vi "Adquisicio_projecte_InsEl (2).vi"() -> ()   [LabVIEW 2014]
uses:
  <vilib>/DAQmx/read.llb/DAQmx Read (Analog 1D Wfm NChan NSamp).vi
  <vilib>/DAQmx/configure/timing.llb/DAQmx Timing (Sample Clock).vi
  <vilib>/DAQmx/miscellaneous.llb/DAQmx Fill In Error Info.vi
panel:
  in  "T alarm max CH 4":dbl
  in  "T alarm min CH 4":dbl
  in  "T alarm max CH 3":dbl
  in  "T alarm min CH 3":dbl
  in  "T alarm min CH 2":dbl
  in  "T alarm max CH 2":dbl
  in  "T alarm max CH 1":dbl
  in  "T alarm min CH 1":dbl
  out "IND CH 4":u32(colorbox)
  out "IND CH 3":u32(colorbox)
  out "IND CH 2":u32(colorbox)
  out "IND CH 1":u32(colorbox)
  in  "V2":dbl
  in  "V1":dbl
  in  "T2":dbl
  in  "T1":dbl
  in  "Numero de Media":dbl
  in  "Durada adquisició(s)":dbl
  in  "Temps entre adquisicions(s)":dbl
  out "?":bool
  out "?":bool
  out "?":bool
  out "?":bool
  in  "CH 4":bool
  in  "CH 3":bool
  in  "CH 2":bool
  in  "CH 1":bool
  in  "?":bool
  in  "?":bool
  out "Registro Temperatura CH 4":dbl(graph)
  out "Registro Temperatura CH 3":dbl(graph)
  out "Registro Temperatura CH 2":dbl(graph)
  out "Registro Temperatura CH 1":dbl(graph)
  in  "Tab Control":enum32{"CH 1", "CH 2", "CH 3", "CH 4"}(tab)
  out "T min CH 1":dbl
  out "T max CH 1":dbl
  out "Desviació 1":dbl
  out "H CH 1":dbl[](array[numeric])
  out "MEDIA CH 1":dbl
  out "Tiempo T max CH1":string
  out "Tiempo T min CH1":string
  out "H CH 2":dbl[](array[numeric])
  out "T max CH 2":dbl
  out "T min CH 2":dbl
  out "Desviació 2":dbl
  out "MEDIA CH 2":dbl
  out "Tiempo T max CH2":string
  out "Tiempo T min CH2":string
  out "H CH 3":dbl[](array[numeric])
  out "T max CH 3":dbl
  out "T min CH 3":dbl
  out "Desviació 3":dbl
  out "MEDIA CH 3":dbl
  out "Tiempo T max CH3":string
  out "Tiempo T min CH3":string
  out "H CH 4":dbl[](array[numeric])
  out "T max CH 4":dbl
  out "T min CH 4":dbl
  out "Desviació 4":dbl
  out "Tiempo T max CH4":string
  out "Tiempo T min CH4":string
  out "MEDIA CH 4":dbl
  # "SISTEMA D'ALARMES"
  # "ACTIVACIÓ CANALS"
  # "CONFIGURACIÓ"
  # "CALIBRATGE"
  # "Temperatura per sobre del màxim"
  # "Temperatura corecta"
  # "Temperatura per sota del mínim"
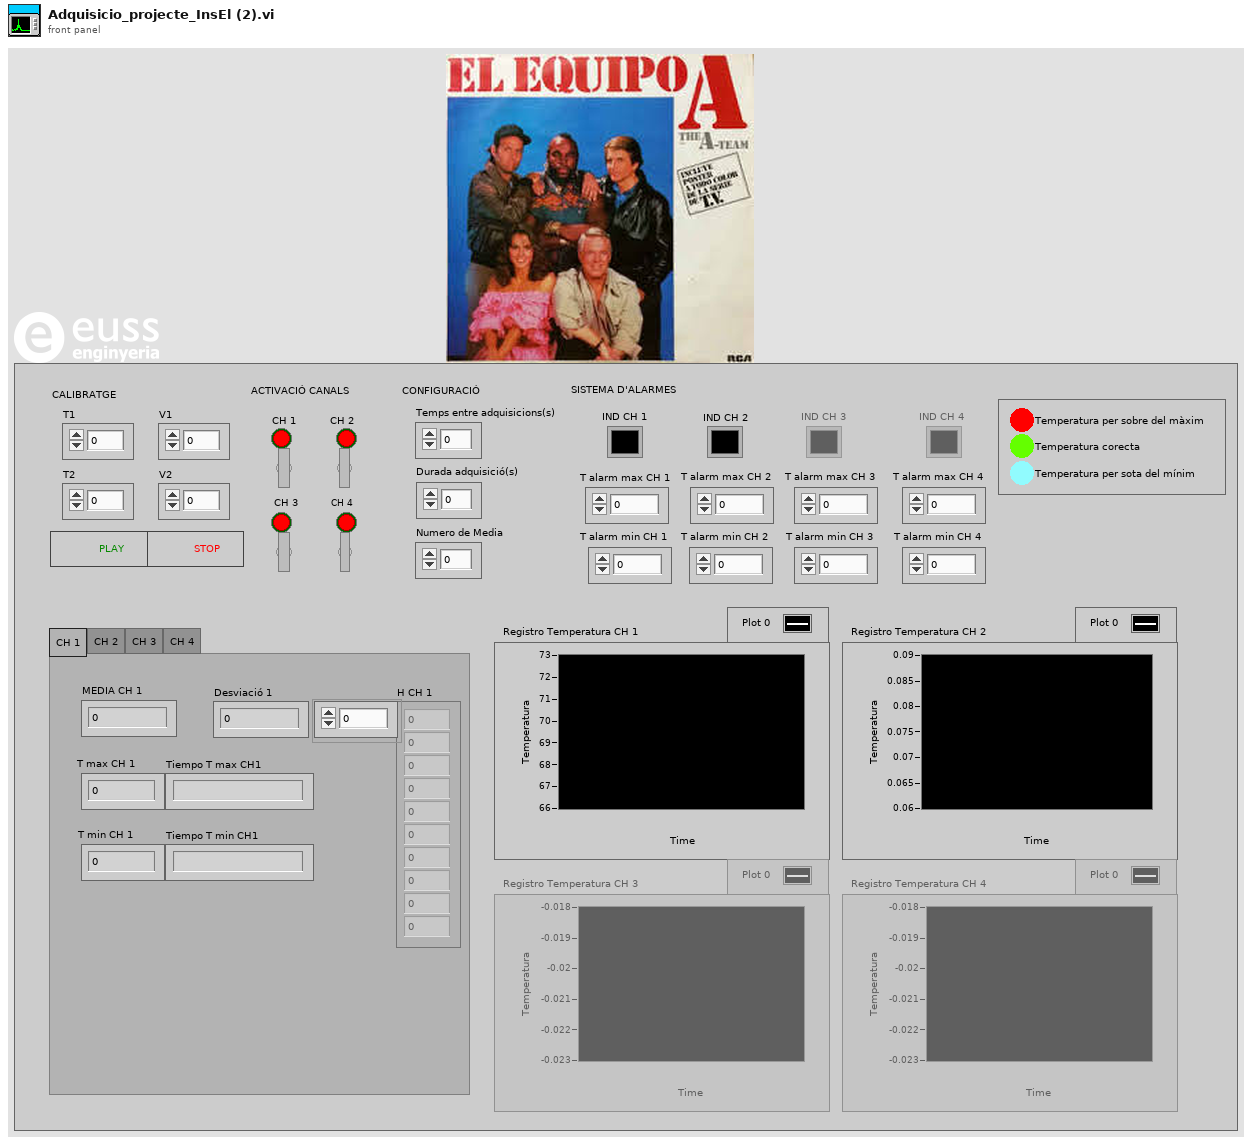
[diagram p1: front panel]
types:
  T1 = enum16{"open", "replace", "create", "open or create", "replace or create", "replace or create with confirmation"}
  T2 = enum8{"Enabled", "Disabled", "Disabled and Grayed Out"}
  T3 = cluster{"CH 1":bool, "CH 2":bool, "CH 3":bool, "CH 4":bool}
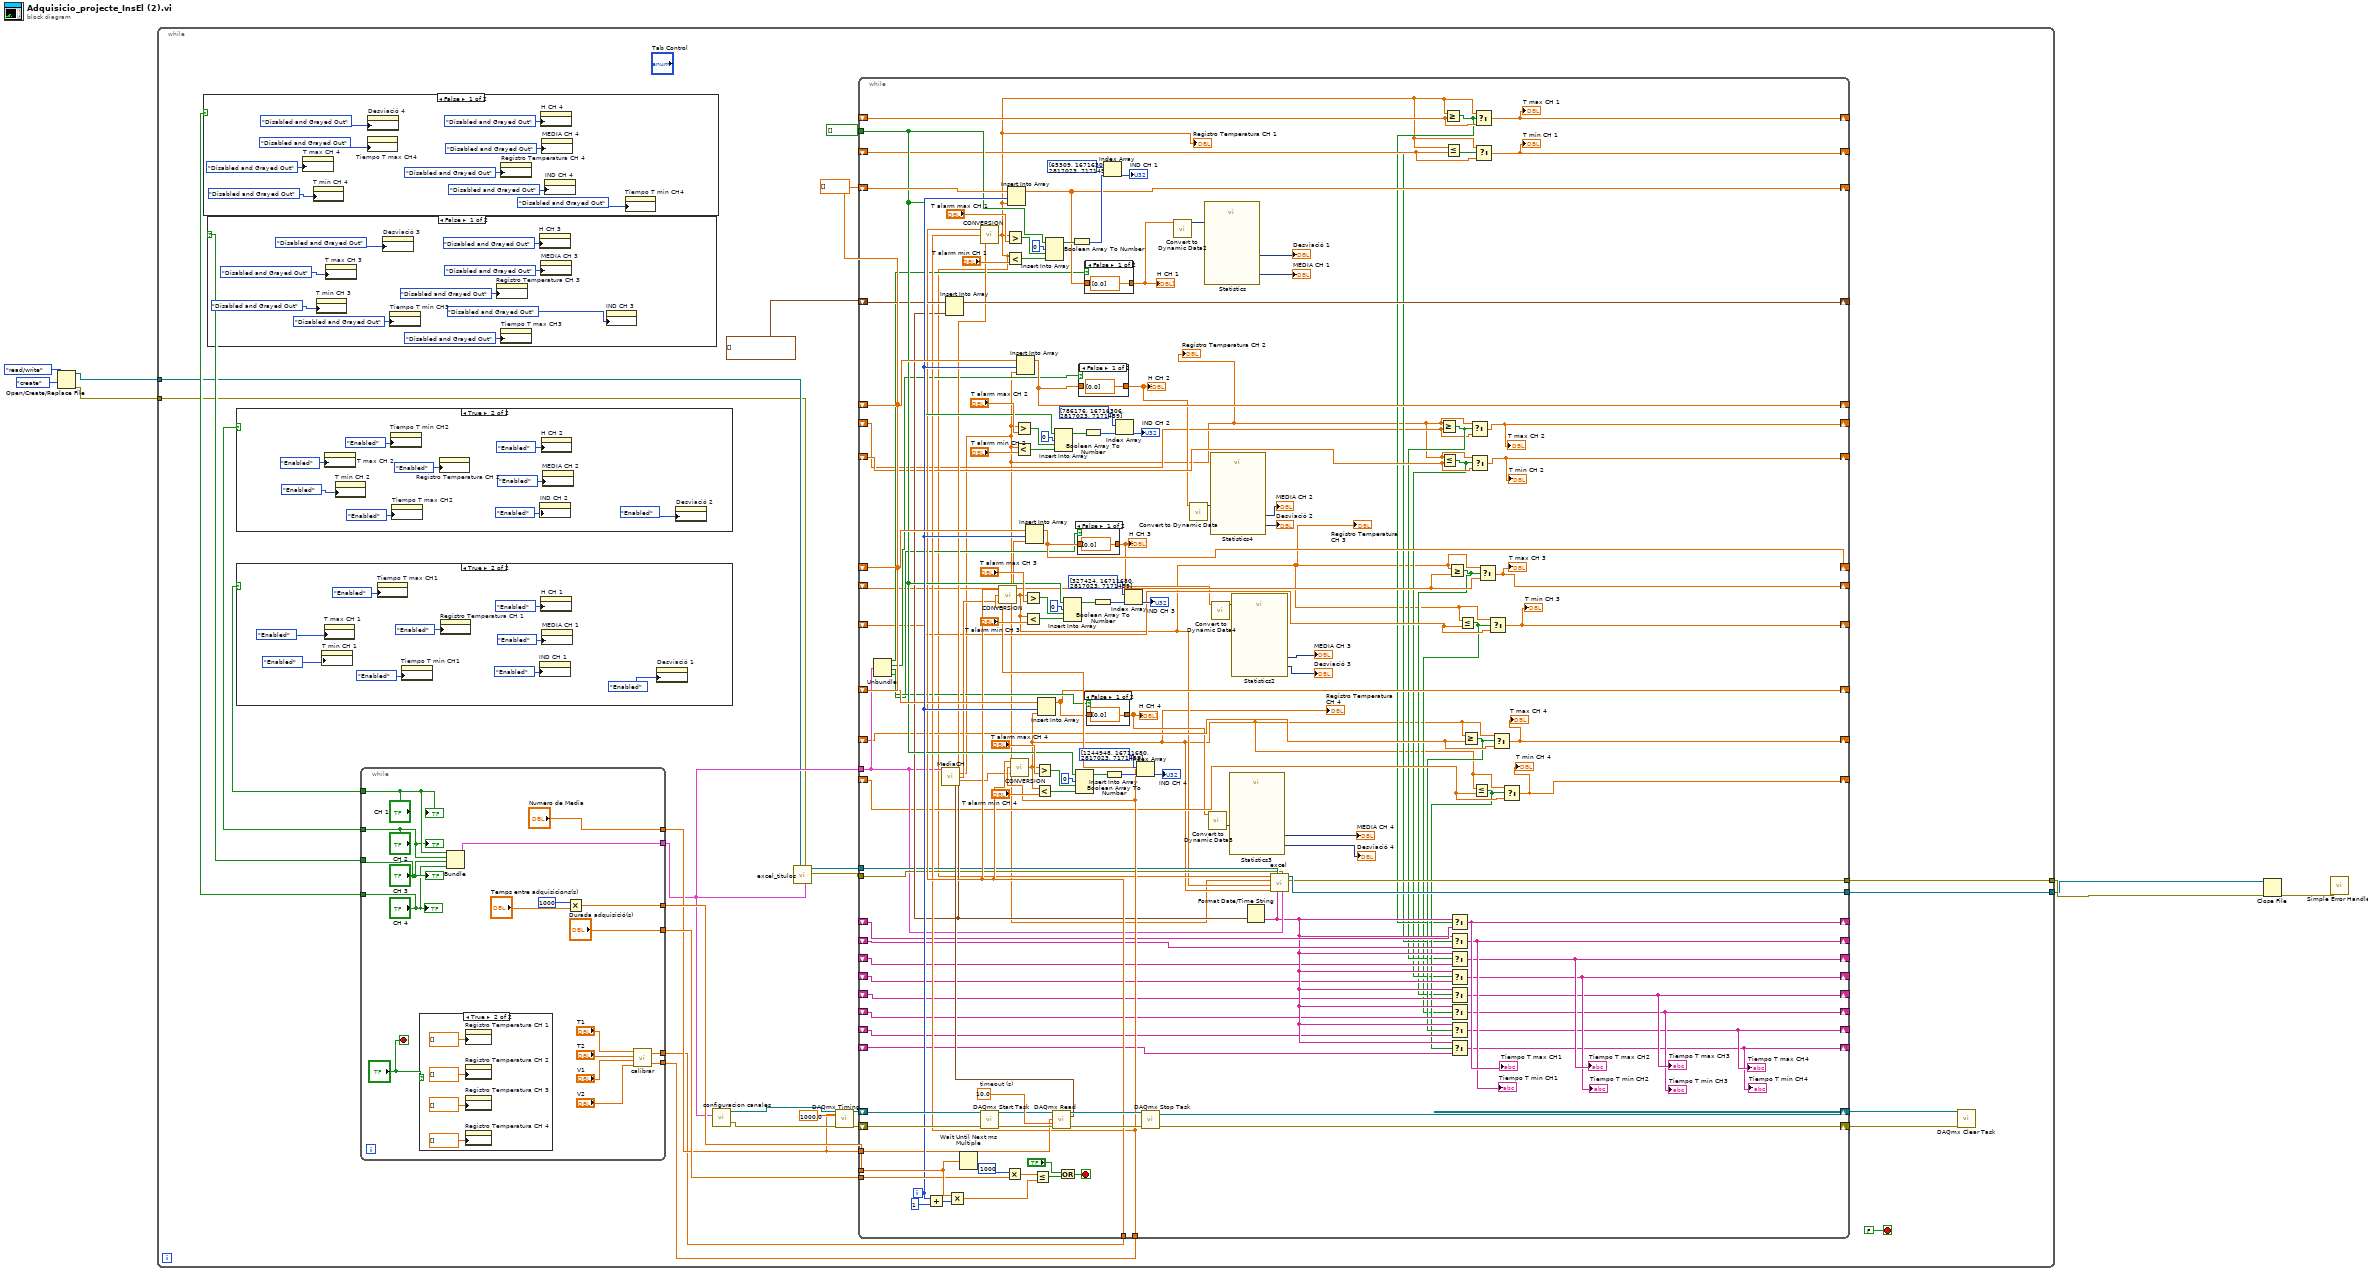
[diagram p0: block diagram]
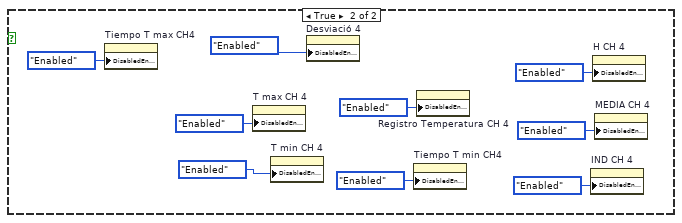
[diagram p2: hidden frame]
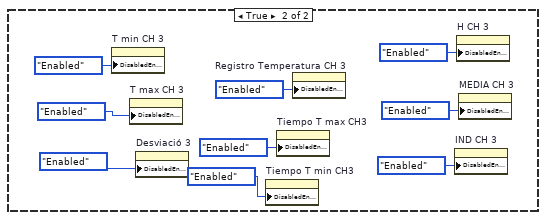
[diagram p3: hidden frame]
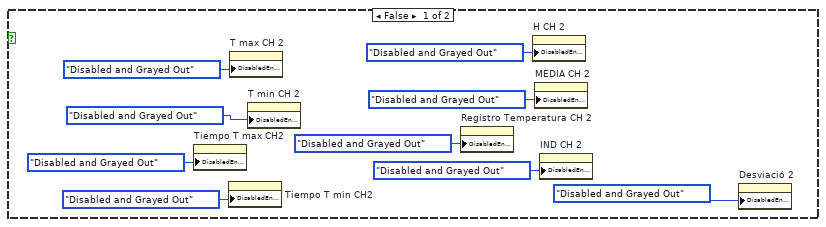
[diagram p4: hidden frame]
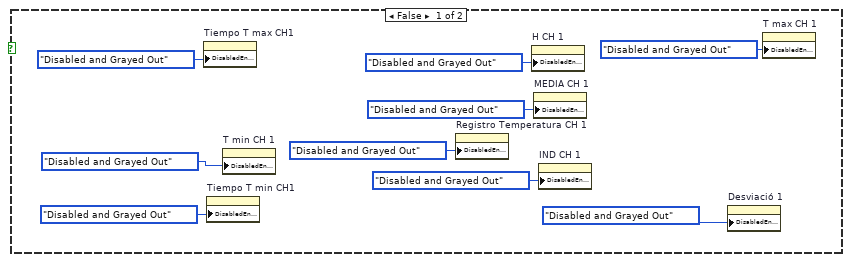
[diagram p5: hidden frame]
diagram:
  n1 = Open/Create/Replace File(operation (0:open)=T1."create", access (0:read/write)=enum16{"read/write", "read-only", "write-only"}."read/write") -> (refnum out=w5:refnum<file>, error out=w4:errorcluster)  [unwired: 4 in, 1 out]
  n2 = while {
    tunnel: w5 -> [w13]
    tunnel: w4 -> [w12]
    tunnel: [w10] -> w2
    tunnel: [w9] -> w1
    stop <- FALSE stop-if-true
    w28 = dbl[] [] ("array")
    n3 = while {
      tunnel: [w123] -> w14
      tunnel: ["CH 1"] -> w26
      tunnel: ["CH 2"] -> w23
      tunnel: ["CH 3"] -> w24
      tunnel: ["CH 4"] -> w25
      tunnel: ["Numero de Media"] -> w19
      tunnel: [w114] -> w21
      tunnel: ["Durada adquisició(s)"] -> w20
      tunnel: [w108] -> w18
      tunnel: [w107] -> w17
      stop <- "?" stop-if-true
      n4 = case shown="True" "?" {
        frame False {
        }
        frame True {
          n5 = property on="Registro Temperatura CH 1" class="WFChart (strict)"("History Data"=dbl[] []) -> ()  [unwired: 2 in, 2 out]
          n6 = property on="Registro Temperatura CH 2" class="WFChart (strict)"("History Data"=dbl[] []) -> ()  [unwired: 2 in, 2 out]
          n7 = property on="Registro Temperatura CH 3" class="WFChart (strict)"("History Data"=dbl[] []) -> ()  [unwired: 2 in, 2 out]
          n8 = property on="Registro Temperatura CH 4" class="WFChart (strict)"("History Data"=dbl[] []) -> ()  [unwired: 2 in, 2 out]
        }
      }
      n9 = Bundle("CH 1"="CH 1", "CH 2"="CH 2", "CH 3"="CH 3", "CH 4"="CH 4") -> (w123:T3)  [unwired: 1 in]
      n10 = Multiply(x=1000, y="Temps entre adquisicions(s)") -> (x*y=w114:dbl)
      n11 = call "calibrar.vi"("V 2"="V2", "V1"="V1", "Temp2"="T2", "Temp"="T1") -> ("B"=w107:dbl, "A"=w108:dbl)
      "?" <- "CH 1"
      "?" <- "CH 2"
      "?" <- "CH 3"
      "?" <- "CH 4"
    }
    n12 = case shown="False" w25 {
      frame False {
        n13 = property on="T max CH 4" class="DigNum (strict)"("DisabledEnum"=T2."Disabled and Grayed Out" ("Disabled")) -> ()  [unwired: 2 in, 2 out]
        n14 = property on="T min CH 4" class="DigNum (strict)"("DisabledEnum"=T2."Disabled and Grayed Out" ("Disabled")) -> ()  [unwired: 2 in, 2 out]
        n15 = property on="Tiempo T max CH4" class="Str"("DisabledEnum"=T2."Disabled and Grayed Out" ("Disabled")) -> ()  [unwired: 2 in, 2 out]
        n16 = property on="Desviació 4" class="DigNum (strict)"("DisabledEnum"=T2."Disabled and Grayed Out" ("Disabled")) -> ()  [unwired: 2 in, 2 out]
        n17 = property on="Registro Temperatura CH 4" class="WFChart (strict)"("DisabledEnum"=T2."Disabled and Grayed Out" ("Disabled")) -> ()  [unwired: 2 in, 2 out]
        n18 = property on="H CH 4" class="Arr (strict)"("DisabledEnum"=T2."Disabled and Grayed Out" ("Disabled")) -> ()  [unwired: 2 in, 2 out]
        n19 = property on="MEDIA CH 4" class="DigNum (strict)"("DisabledEnum"=T2."Disabled and Grayed Out" ("Disabled")) -> ()  [unwired: 2 in, 2 out]
        n20 = property on="IND CH 4" class="ColBox"("DisabledEnum"=T2."Disabled and Grayed Out" ("Disabled")) -> ()  [unwired: 2 in, 2 out]
        n21 = property on="Tiempo T min CH4" class="Str"("DisabledEnum"=T2."Disabled and Grayed Out" ("Disabled")) -> ()  [unwired: 2 in, 2 out]
      }
      frame True {
        n22 = property on="Tiempo T max CH4" class="Str"("DisabledEnum"=T2."Enabled" ("Disabled")) -> ()  [unwired: 2 in, 2 out]
        n23 = property on="T max CH 4" class="DigNum (strict)"("DisabledEnum"=T2."Enabled" ("Disabled")) -> ()  [unwired: 2 in, 2 out]
        n24 = property on="T min CH 4" class="DigNum (strict)"("DisabledEnum"=T2."Enabled" ("Disabled")) -> ()  [unwired: 2 in, 2 out]
        n25 = property on="Desviació 4" class="DigNum (strict)"("DisabledEnum"=T2."Enabled" ("Disabled")) -> ()  [unwired: 2 in, 2 out]
        n26 = property on="Tiempo T min CH4" class="Str"("DisabledEnum"=T2."Enabled" ("Disabled")) -> ()  [unwired: 2 in, 2 out]
        n27 = property on="Registro Temperatura CH 4" class="WFChart (strict)"("DisabledEnum"=T2."Enabled" ("Disabled")) -> ()  [unwired: 2 in, 2 out]
        n28 = property on="IND CH 4" class="ColBox"("DisabledEnum"=T2."Enabled" ("Disabled")) -> ()  [unwired: 2 in, 2 out]
        n29 = property on="H CH 4" class="Arr (strict)"("DisabledEnum"=T2."Enabled" ("Disabled")) -> ()  [unwired: 2 in, 2 out]
        n30 = property on="MEDIA CH 4" class="DigNum (strict)"("DisabledEnum"=T2."Enabled" ("Disabled")) -> ()  [unwired: 2 in, 2 out]
      }
    }
    n31 = case shown="False" w24 {
      frame False {
        n32 = property on="T min CH 3" class="DigNum (strict)"("DisabledEnum"=T2."Disabled and Grayed Out" ("Disabled")) -> ()  [unwired: 2 in, 2 out]
        n33 = property on="T max CH 3" class="DigNum (strict)"("DisabledEnum"=T2."Disabled and Grayed Out" ("Disabled")) -> ()  [unwired: 2 in, 2 out]
        n34 = property on="Desviació 3" class="DigNum (strict)"("DisabledEnum"=T2."Disabled and Grayed Out" ("Disabled")) -> ()  [unwired: 2 in, 2 out]
        n35 = property on="Tiempo T min CH3" class="Str"("DisabledEnum"=T2."Disabled and Grayed Out" ("Disabled")) -> ()  [unwired: 2 in, 2 out]
        n36 = property on="Registro Temperatura CH 3" class="WFChart (strict)"("DisabledEnum"=T2."Disabled and Grayed Out" ("Disabled")) -> ()  [unwired: 2 in, 2 out]
        n37 = property on="Tiempo T max CH3" class="Str"("DisabledEnum"=T2."Disabled and Grayed Out" ("Disabled")) -> ()  [unwired: 2 in, 2 out]
        n38 = property on="H CH 3" class="Arr (strict)"("DisabledEnum"=T2."Disabled and Grayed Out" ("Disabled")) -> ()  [unwired: 2 in, 2 out]
        n39 = property on="MEDIA CH 3" class="DigNum (strict)"("DisabledEnum"=T2."Disabled and Grayed Out" ("Disabled")) -> ()  [unwired: 2 in, 2 out]
        n40 = property on="IND CH 3" class="ColBox"("DisabledEnum"=T2."Disabled and Grayed Out" ("Disabled")) -> ()  [unwired: 2 in, 2 out]
      }
      frame True {
        n41 = property on="T min CH 3" class="DigNum (strict)"("DisabledEnum"=T2."Enabled" ("Disabled")) -> ()  [unwired: 2 in, 2 out]
        n42 = property on="T max CH 3" class="DigNum (strict)"("DisabledEnum"=T2."Enabled" ("Disabled")) -> ()  [unwired: 2 in, 2 out]
        n43 = property on="Desviació 3" class="DigNum (strict)"("DisabledEnum"=T2."Enabled" ("Disabled")) -> ()  [unwired: 2 in, 2 out]
        n44 = property on="Tiempo T min CH3" class="Str"("DisabledEnum"=T2."Enabled" ("Disabled")) -> ()  [unwired: 2 in, 2 out]
        n45 = property on="Tiempo T max CH3" class="Str"("DisabledEnum"=T2."Enabled" ("Disabled")) -> ()  [unwired: 2 in, 2 out]
        n46 = property on="Registro Temperatura CH 3" class="WFChart (strict)"("DisabledEnum"=T2."Enabled" ("Disabled")) -> ()  [unwired: 2 in, 2 out]
        n47 = property on="IND CH 3" class="ColBox"("DisabledEnum"=T2."Enabled" ("Disabled")) -> ()  [unwired: 2 in, 2 out]
        n48 = property on="H CH 3" class="Arr (strict)"("DisabledEnum"=T2."Enabled" ("Disabled")) -> ()  [unwired: 2 in, 2 out]
        n49 = property on="MEDIA CH 3" class="DigNum (strict)"("DisabledEnum"=T2."Enabled" ("Disabled")) -> ()  [unwired: 2 in, 2 out]
      }
    }
    n50 = case shown="True" w23 {
      frame False {
        n51 = property on="Tiempo T max CH2" class="Str"("DisabledEnum"=T2."Disabled and Grayed Out" ("Disabled")) -> ()  [unwired: 2 in, 2 out]
        n52 = property on="Tiempo T min CH2" class="Str"("DisabledEnum"=T2."Disabled and Grayed Out" ("Disabled")) -> ()  [unwired: 2 in, 2 out]
        n53 = property on="T max CH 2" class="DigNum (strict)"("DisabledEnum"=T2."Disabled and Grayed Out" ("Disabled")) -> ()  [unwired: 2 in, 2 out]
        n54 = property on="T min CH 2" class="DigNum (strict)"("DisabledEnum"=T2."Disabled and Grayed Out" ("Disabled")) -> ()  [unwired: 2 in, 2 out]
        n55 = property on="Registro Temperatura CH 2" class="WFChart (strict)"("DisabledEnum"=T2."Disabled and Grayed Out" ("Disabled")) -> ()  [unwired: 2 in, 2 out]
        n56 = property on="H CH 2" class="Arr (strict)"("DisabledEnum"=T2."Disabled and Grayed Out" ("Disabled")) -> ()  [unwired: 2 in, 2 out]
        n57 = property on="MEDIA CH 2" class="DigNum (strict)"("DisabledEnum"=T2."Disabled and Grayed Out" ("Disabled")) -> ()  [unwired: 2 in, 2 out]
        n58 = property on="IND CH 2" class="ColBox"("DisabledEnum"=T2."Disabled and Grayed Out" ("Disabled")) -> ()  [unwired: 2 in, 2 out]
        n59 = property on="Desviació 2" class="DigNum (strict)"("DisabledEnum"=T2."Disabled and Grayed Out" ("Disabled")) -> ()  [unwired: 2 in, 2 out]
      }
      frame True {
        n60 = property on="T max CH 2" class="DigNum (strict)"("DisabledEnum"=T2."Enabled" ("Disabled")) -> ()  [unwired: 2 in, 2 out]
        n61 = property on="T min CH 2" class="DigNum (strict)"("DisabledEnum"=T2."Enabled" ("Disabled")) -> ()  [unwired: 2 in, 2 out]
        n62 = property on="Tiempo T min CH2" class="Str"("DisabledEnum"=T2."Enabled" ("Disabled")) -> ()  [unwired: 2 in, 2 out]
        n63 = property on="Tiempo T max CH2" class="Str"("DisabledEnum"=T2."Enabled" ("Disabled")) -> ()  [unwired: 2 in, 2 out]
        n64 = property on="Registro Temperatura CH 2" class="WFChart (strict)"("DisabledEnum"=T2."Enabled" ("Disabled")) -> ()  [unwired: 2 in, 2 out]
        n65 = property on="IND CH 2" class="ColBox"("DisabledEnum"=T2."Enabled" ("Disabled")) -> ()  [unwired: 2 in, 2 out]
        n66 = property on="H CH 2" class="Arr (strict)"("DisabledEnum"=T2."Enabled" ("Disabled")) -> ()  [unwired: 2 in, 2 out]
        n67 = property on="MEDIA CH 2" class="DigNum (strict)"("DisabledEnum"=T2."Enabled" ("Disabled")) -> ()  [unwired: 2 in, 2 out]
        n68 = property on="Desviació 2" class="DigNum (strict)"("DisabledEnum"=T2."Enabled" ("Disabled")) -> ()  [unwired: 2 in, 2 out]
      }
    }
    n69 = case shown="True" w26 {
      frame False {
        n70 = property on="Tiempo T max CH1" class="Str"("DisabledEnum"=T2."Disabled and Grayed Out" ("Disabled")) -> ()  [unwired: 2 in, 2 out]
        n71 = property on="Tiempo T min CH1" class="Str"("DisabledEnum"=T2."Disabled and Grayed Out" ("Disabled")) -> ()  [unwired: 2 in, 2 out]
        n72 = property on="T min CH 1" class="DigNum (strict)"("DisabledEnum"=T2."Disabled and Grayed Out" ("Disabled")) -> ()  [unwired: 2 in, 2 out]
        n73 = property on="Registro Temperatura CH 1" class="WFChart (strict)"("DisabledEnum"=T2."Disabled and Grayed Out" ("Disabled")) -> ()  [unwired: 2 in, 2 out]
        n74 = property on="H CH 1" class="Arr (strict)"("DisabledEnum"=T2."Disabled and Grayed Out" ("Disabled")) -> ()  [unwired: 2 in, 2 out]
        n75 = property on="MEDIA CH 1" class="DigNum (strict)"("DisabledEnum"=T2."Disabled and Grayed Out" ("Disabled")) -> ()  [unwired: 2 in, 2 out]
        n76 = property on="IND CH 1" class="ColBox"("DisabledEnum"=T2."Disabled and Grayed Out" ("Disabled")) -> ()  [unwired: 2 in, 2 out]
        n77 = property on="Desviació 1" class="DigNum (strict)"("DisabledEnum"=T2."Disabled and Grayed Out" ("Disabled")) -> ()  [unwired: 2 in, 2 out]
        n78 = property on="T max CH 1" class="DigNum (strict)"("DisabledEnum"=T2."Disabled and Grayed Out" ("Disabled")) -> ()  [unwired: 2 in, 2 out]
      }
      frame True {
        n79 = property on="T min CH 1" class="DigNum (strict)"("DisabledEnum"=T2."Enabled" ("Disabled")) -> ()  [unwired: 2 in, 2 out]
        n80 = property on="T max CH 1" class="DigNum (strict)"("DisabledEnum"=T2."Enabled" ("Disabled")) -> ()  [unwired: 2 in, 2 out]
        n81 = property on="Tiempo T max CH1" class="Str"("DisabledEnum"=T2."Enabled" ("Disabled")) -> ()  [unwired: 2 in, 2 out]
        n82 = property on="Tiempo T min CH1" class="Str"("DisabledEnum"=T2."Enabled" ("Disabled")) -> ()  [unwired: 2 in, 2 out]
        n83 = property on="Registro Temperatura CH 1" class="WFChart (strict)"("DisabledEnum"=T2."Enabled" ("Disabled")) -> ()  [unwired: 2 in, 2 out]
        n84 = property on="IND CH 1" class="ColBox"("DisabledEnum"=T2."Enabled" ("Disabled")) -> ()  [unwired: 2 in, 2 out]
        n85 = property on="H CH 1" class="Arr (strict)"("DisabledEnum"=T2."Enabled" ("Disabled")) -> ()  [unwired: 2 in, 2 out]
        n86 = property on="MEDIA CH 1" class="DigNum (strict)"("DisabledEnum"=T2."Enabled" ("Disabled")) -> ()  [unwired: 2 in, 2 out]
        n87 = property on="Desviació 1" class="DigNum (strict)"("DisabledEnum"=T2."Enabled" ("Disabled")) -> ()  [unwired: 2 in, 2 out]
      }
    }
    n88 = call "configuracion canales.vi"("input cluster"=w14) -> ("error out"=w30:errorcluster, "task out"=w8:refnum<k21>)  [unwired: 3 in]
    n89 = call "excel_titulos.vi"("input cluster"=w14, "error out"=w12, "refnum out"=w13) -> ("error in"=w15:errorcluster, "refnum"=w16:refnum<file>)  [unwired: 7 in]
    n90 = call-poly <vilib>:"DAQmx Timing.vi"("task/channels in"=w8, "samples per channel"=w19, "rate"=1000.0, "error in"=w30) -> ("task out"=w32:refnum<k21>, "error out"=w31:errorcluster)  [unwired: 10 in]
    n91 = while {
      shift-right: [w269] -> w34
      shift-left: w32 -> [w265]
      shift-right: [w268] -> w33
      shift-left: w31 -> [w255]
      tunnel: w21 -> [w259]
      tunnel: w14 -> [w186]
      tunnel: w19 -> [w211]
      tunnel: w20 -> [w256]
      shift-right: [w180] -> _
      shift-left: w28 -> [w253]
      shift-right: [w182] -> _
      shift-left: w28 -> [w252]
      shift-right: [w184] -> _
      shift-left: w28 -> [w251]
      shift-right: [w178] -> _
      shift-left: w28 -> [w249]
      tunnel: bool[] [] ("array") -> [w216]
      shift-right: [w208] -> _
      shift-left: timestamp[] [] ("array") -> [w209]
      tunnel: w18 -> [w207]
      tunnel: w17 -> [w206]
      tunnel: [w196] -> w9
      tunnel: [w195] -> w10
      tunnel: w16 -> [w194]
      tunnel: w15 -> [w193]
      shift-right: [w176] -> _
      shift-left: _ -> [w177]
      shift-right: [w175] -> _
      shift-left: _ -> [w174]
      shift-right: [w163] -> _
      shift-left: _ -> [w173]
      shift-right: [w147] -> _
      shift-left: _ -> [w171]
      shift-right: [w146] -> _
      shift-left: _ -> [w169]
      shift-right: [w145] -> _
      shift-left: _ -> [w168]
      shift-right: [w144] -> _
      shift-left: _ -> [w167]
      shift-right: [w143] -> _
      shift-left: _ -> [w166]
      shift-right: [w142] -> _
      shift-left: _ -> [w165]
      shift-right: [w141] -> _
      shift-left: _ -> [w164]
      shift-right: [w157] -> _
      shift-left: _ -> [w158]
      shift-right: [w160] -> _
      shift-left: _ -> [w159]
      shift-right: [w155] -> _
      shift-left: _ -> [w131]
      shift-right: [w154] -> _
      shift-left: _ -> [w156]
      shift-right: [w151] -> _
      shift-left: _ -> [w153]
      shift-right: [w150] -> _
      shift-left: _ -> [w152]
      i -> [w250]
      stop <- w257 stop-if-true
      w272 = 10.0  # timeout (s)
      n92 = Unbundle(w186) -> ("CH 1"=w179:bool, "CH 2"=w181:bool, "CH 3"=w183:bool, "CH 4"=w185:bool)
      n93 = Add(x=w250, y=1 ("x")) -> (x+y=w258:i32)
      n94 = Multiply(x=w259, y=w258) -> (x*y=w260:dbl)
      n95 = Wait Until Next ms Multiple(millisecond multiple=w259) -> ()  [unwired: 1 out]
      n96 = call <vilib>:"DAQmx Start Task.vi"("task/channels in"=w265, "error in"=w255) -> ("task out"=w270:refnum<k21>, "error out"=w271:errorcluster)  [unwired: 12 in]
      n97 = Multiply(x=1000, y=w256) -> (x*y=w262:dbl)
      n98 = Less Or Equal?(x=w262, y=w260) -> (x <= y?=w261:bool)
      n99 = call-poly <vilib>:"DAQmx Read.vi"("task/channels in"=w270, "number of samples per channel"=w211, "timeout"=w272, "error in"=w271) -> ("task out"=w267:refnum<k21>, "data"=w210:waveform(dbl)[], "error out"=w266:errorcluster)  [unwired: 9 in]
      n100 = call "MediaCH.vi"("input cluster"=w186, "Data"=w210) -> ("Mitja CH1"=w203:dbl, "Mitja CH2"=w128:dbl, "Mitja CH3"=w204:dbl, "Mitja CH4"=w205:dbl, "Time Stamp"=w197:timestamp)  [unwired: 9 in]
      "Registro Temperatura CH 2" <- w128
      n101 = Insert Into Array(array=w209, new element=w197) -> (w208:timestamp[])  [unwired: 1 in]
      n102 = call "CONVERSION.vi"("V1"=w203, "B"=w206, "A"=w207) -> ("Temp"=w132:dbl)
      "Registro Temperatura CH 1" <- w132
      n103 = call "CONVERSION.vi"("V1"=w204, "B"=w206, "A"=w207) -> ("Temp"=w130:dbl)
      "Registro Temperatura CH 3" <- w130
      n104 = Greater?(x=w132, y="T alarm max CH 1") -> (0:w246:bool)
      n105 = Less?(x=w132, y="T alarm min CH 1") -> (x < y?=w245:bool)
      n106 = Insert Into Array(array=w253, index=w250, new element=w132) -> (w180:dbl[])
      n107 = call "CONVERSION.vi"("V1"=w205, "B"=w206, "A"=w207) -> ("Temp"=w129:dbl)
      "Registro Temperatura CH 4" <- w129
      n108 = Greater?(x=w128, y="T alarm max CH 2") -> (0:w238:bool)
      n109 = Less?(x=w128, y="T alarm min CH 2") -> (x < y?=w237:bool)
      n110 = Insert Into Array(array=w252, index=w250, new element=w128) -> (w182:dbl[])
      n111 = Greater?(x=w130, y="T alarm max CH 3") -> (0:w231:bool)
      n112 = Less?(x=w130, y="T alarm min CH 3") -> (x < y?=w230:bool)
      n113 = Insert Into Array(array=w251, index=w250, new element=w130) -> (w184:dbl[])
      n114 = Greater?(x=w129, y="T alarm max CH 4") -> (0:w223:bool)
      n115 = Less?(x=w129, y="T alarm min CH 4") -> (x < y?=w222:bool)
      n116 = Insert Into Array(array=w249, index=w250, new element=w129) -> (w178:dbl[])
      n117 = Insert Into Array(array=w216, index=0, new element #1=w246, new element #2=w245) -> (w243:bool[])
      n118 = Insert Into Array(array=w216, index=0, new element #1=w238, new element #2=w237) -> (w235:bool[])
      n119 = Or(x="?", y=w261) -> (x .or. y?=w257:bool)
      n120 = Insert Into Array(array=w216, index=0, new element #1=w231, new element #2=w230) -> (w228:bool[])
      n121 = Boolean Array To Number(Boolean array=w243) -> (number=w241:u32)
      n122 = Insert Into Array(array=w216, index=0, new element #1=w223, new element #2=w222) -> (w220:bool[])
      n123 = case shown="False" w183 {
        tunnel: w184 -> [_ w278]
        tunnel: [dbl[] [0.0] ("array") w278] -> w134
        frame False {
        }
        frame True {
        }
      }
      "H CH 3" <- w134
      n124 = case shown="False" w181 {
        tunnel: w182 -> [_ w276]
        tunnel: [dbl[] [0.0] ("array") w276] -> w135
        frame False {
        }
        frame True {
        }
      }
      "H CH 2" <- w135
      n125 = case shown="False" w179 {
        tunnel: w180 -> [_ w274]
        tunnel: [dbl[] [0.0] ("array") w274] -> w136
        frame False {
        }
        frame True {
        }
      }
      "H CH 1" <- w136
      n126 = Boolean Array To Number(Boolean array=w235) -> (number=w233:u32)
      n127 = case shown="False" w185 {
        tunnel: w178 -> [_ w280]
        tunnel: [dbl[] [0.0] ("array") w280] -> w133
        frame False {
        }
        frame True {
        }
      }
      "H CH 4" <- w133
      n128 = Boolean Array To Number(Boolean array=w228) -> (number=w226:u32)
      n129 = Index Array(array=u32[] [65309, 16716306, 2817023, 7171459], index=w241) -> (element=→"IND CH 1":u32)
      n130 = Boolean Array To Number(Boolean array=w220) -> (number=w217:u32)
      n131 = Index Array(array=u32[] [786176, 16716306, 2817023, 7171459], index=w233) -> (element=→"IND CH 2":u32)
      n132 = Index Array(array=u32[] [327424, 16711680, 2817023, 7171459], index=w226) -> (element=→"IND CH 3":u32)
      n133 = Index Array(array=u32[] [1244948, 16711680, 2817023, 7171459], index=w217) -> (element=→"IND CH 4":u32)
      n134 = call <vilib>:"DAQmx Stop Task.vi"("task/channels in"=w267, "error in"=w266) -> ("task out"=w269:refnum<k21>, "error out"=w268:errorcluster)  [unwired: 12 in]
      n135 = call "Convert to Dynamic Data2"("Array"=w136) -> ("Dynamic Data Type"=w200:dynamicdata)  [unwired: 3 in]
      n136 = call "Convert to Dynamic Data"("Array"=w135) -> ("Dynamic Data Type"=w192:dynamicdata)  [unwired: 3 in]
      n137 = call "Statistics"("Signals"=w200) -> ("Standard Dev"=→"Desviació 1":dynamicdata, "Arithmetic Mean"=→"MEDIA CH 1":dynamicdata)  [unwired: 20 in, 5 out]
      n138 = call "Convert to Dynamic Data5"("Array"=w133) -> ("Dynamic Data Type"=w198:dynamicdata)  [unwired: 3 in]
      n139 = call "Statistics4"("Signals"=w192) -> ("Standard Dev"=→"Desviació 2":dynamicdata, "Arithmetic Mean"=→"MEDIA CH 2":dynamicdata)  [unwired: 20 in, 5 out]
      n140 = call "Convert to Dynamic Data4"("Array"=w134) -> ("Dynamic Data Type"=w199:dynamicdata)  [unwired: 3 in]
      n141 = call "Statistics3"("Signals"=w198) -> ("Standard Dev"=→"Desviació 4":dynamicdata, "Arithmetic Mean"=→"MEDIA CH 4":dynamicdata)  [unwired: 20 in, 5 out]
      n142 = call "Statistics2"("Signals"=w199) -> ("Standard Dev"=→"Desviació 3":dynamicdata, "Arithmetic Mean"=→"MEDIA CH 3":dynamicdata)  [unwired: 20 in, 5 out]
      n143 = Format Date/Time String(seconds (now)=w197) -> (date/time string=w170:string)  [unwired: 2 in]
      n144 = call "excel.vi"("input cluster"=w186, "error out"=w193, "fecha y hora"=w170, "refnum out"=w194, "CH 4"=w129, "CH 3"=w130, "CH 2"=w128, "CH 1"=w132) -> ("error in"=w195:errorcluster, "refnum"=w196:refnum<file>)  [unwired: 2 in]
      n145 = Greater Or Equal?(x=w128, y=w131) -> (x >= y?=w140:bool)
      n146 = Less Or Equal?(x=w128, y=w156) -> (x <= y?=w139:bool)
      n147 = Greater Or Equal?(x=w132, y=w153) -> (x >= y?=w149:bool)
      n148 = Less Or Equal?(x=w132, y=w152) -> (x <= y?=w148:bool)
      n149 = Greater Or Equal?(x=w130, y=w159) -> (x >= y?=w138:bool)
      n150 = Select(t=w170, s=w149, f=w174) -> (s? t:f=w175:string)
      "Tiempo T max CH1" <- w175
      n151 = Select(t=w170, s=w148, f=w171) -> (s? t:f=w147:string)
      "Tiempo T min CH1" <- w147
      n152 = Select(t=w170, s=w140, f=w169) -> (s? t:f=w146:string)
      "Tiempo T max CH2" <- w146
      n153 = Select(t=w170, s=w139, f=w168) -> (s? t:f=w145:string)
      "Tiempo T min CH2" <- w145
      n154 = Select(t=w170, s=w138, f=w167) -> (s? t:f=w144:string)
      "Tiempo T max CH3" <- w144
      n155 = Less Or Equal?(x=w130, y=w158) -> (x <= y?=w137:bool)
      n156 = Select(t=w170, s=w137, f=w166) -> (s? t:f=w143:string)
      "Tiempo T min CH3" <- w143
      n157 = Greater Or Equal?(x=w129, y=w177) -> (x >= y?=w162:bool)
      n158 = Select(t=w170, s=w162, f=w165) -> (s? t:f=w142:string)
      "Tiempo T max CH4" <- w142
      n159 = Select(t=w128, s=w140, f=w131) -> (s? t:f=w155:dbl)
      "T max CH 2" <- w155
      n160 = Select(t=w128, s=w139, f=w156) -> (s? t:f=w154:dbl)
      "T min CH 2" <- w154
      n161 = Less Or Equal?(x=w129, y=w173) -> (x <= y?=w161:bool)
      n162 = Select(t=w170, s=w161, f=w164) -> (s? t:f=w141:string)
      "Tiempo T min CH4" <- w141
      n163 = Select(t=w132, s=w149, f=w153) -> (s? t:f=w151:dbl)
      "T max CH 1" <- w151
      n164 = Select(t=w132, s=w148, f=w152) -> (s? t:f=w150:dbl)
      "T min CH 1" <- w150
      n165 = Select(t=w130, s=w138, f=w159) -> (s? t:f=w160:dbl)
      "T max CH 3" <- w160
      n166 = Select(t=w130, s=w137, f=w158) -> (s? t:f=w157:dbl)
      "T min CH 3" <- w157
      n167 = Select(t=w129, s=w162, f=w177) -> (s? t:f=w176:dbl)
      "T max CH 4" <- w176
      n168 = Select(t=w129, s=w161, f=w173) -> (s? t:f=w163:dbl)
      "T min CH 4" <- w163
    }
    n169 = call <vilib>:"DAQmx Clear Task.vi"("task in"=w34, "error in"=w33) -> ()  [unwired: 13 in, 1 out]
  }
  n170 = Close File(refnum=w1, error in=w2) -> (error out=w3:errorcluster)  [unwired: 1 out]
  n171 = call <vilib>:"Simple Error Handler.vi"("error in (no error)"=w3) -> ()  [unwired: 4 in, 5 out]
